vi "Constant Curvature Drive.vi"(8 "Turbo?":bool, 9 "QuickTurn?":bool, 10 "Speed":dbl(slide) scale=-1.0..1.0, 11 "Curve":dbl(slide) scale=-1.0..1.0) -> (0 "Right Percent Setpoint":dbl, 3 "Left Percent Setpoint":dbl)   [LabVIEW 2018]
uses:
  <vilib>/Rock Robotics/WPI/Joystick/WPI_JoystickRatioCurveMapping.vi
panel:
  in  "Turbo Max %Output":dbl=0.9
  in  "Deadband":dbl=0.025
  in  "Sensitivity":dbl=0.1
  in  "Normal Max %Output":dbl=0.7
  # "Drive like a car, where any turning input will yield the same curve, regardless of the speed it is traveled at\nUse Velocity PIDF with these outputs, it fights turning over shoot and makes you drive straight\n1718 said to do these things but 4810 put it into code"
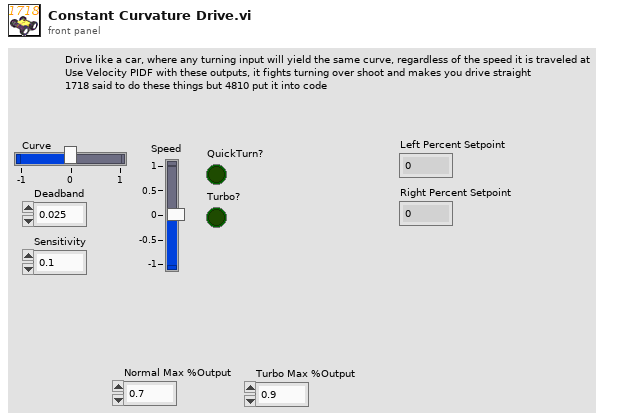
[diagram p1: front panel]
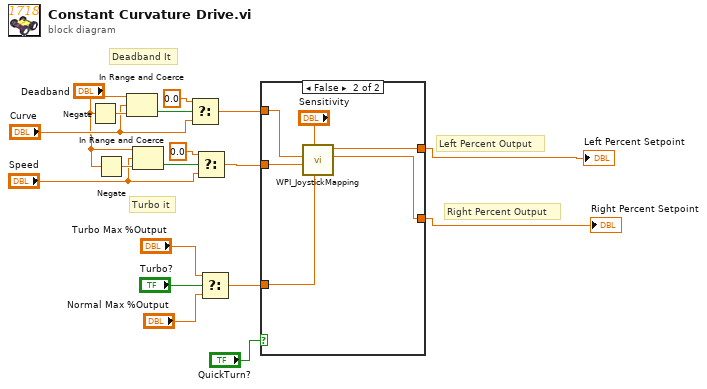
[diagram p0: block diagram]
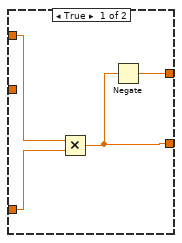
[diagram p2: hidden frame]
diagram:
  # "Right Percent Output"
  # "Left Percent Output"
  # "Turbo it"
  # "Deadband It"
  n1 = Negate(x="Deadband") -> (-x=w16:dbl)
  n2 = Negate(x="Deadband") -> (-x=w14:dbl)
  n3 = In Range and Coerce(upper limit="Deadband", x="Curve", lower limit=w16) -> (In Range?=w18:bool)  [unwired: 1 out]
  n4 = In Range and Coerce(upper limit="Deadband", x="Speed", lower limit=w14) -> (In Range?=w12:bool)  [unwired: 1 out]
  n5 = Select(t=0.0 ("Default Value"), s=w18, f="Curve") -> (s? t:f=w9:dbl)
  n6 = Select(t=0.0 ("Default Value"), s=w12, f="Speed") -> (s? t:f=w8:dbl)
  n7 = Select(t="Turbo Max %Output", s="Turbo?", f="Normal Max %Output") -> (s? t:f=w4:dbl)
  n8 = case shown="False" "QuickTurn?" {
    tunnel: w9 -> [w22 w28]
    tunnel: w8 -> [_ w27]
    tunnel: w4 -> [w21 w25]
    tunnel: [w19 w24] -> w2
    tunnel: [w20 w23] -> w1
    frame True {
      n9 = Multiply(x=w22, y=w21) -> (x*y=w20:dbl)
      n10 = Negate(x=w20) -> (-x=w19:dbl)
    }
    frame False {
      n11 = call-poly <vilib>:"WPI_JoystickMapping.vi"("Max Output"=w25, "Sensitivity"="Sensitivity", "Y axis value (Speed)"=w27, "X axis value (Curve)"=w28) -> ("Right Motor Value"=w23:dbl, "Left Motor Value"=w24:dbl)  [unwired: 6 in]
    }
  }
  "Left Percent Setpoint" <- w2
  "Right Percent Setpoint" <- w1
